vi "extract_offset.vi"(8 "error in (no error)":errorcluster, 10 "xml header string":string, 11 "xpaths":T1) -> (0 "error out":errorcluster, 3 "offset":refnum<class "SpaceVector.lvclass">)   [LabVIEW 2010, in "XImage.xctl"]
uses:
  XImage.xctl
  xpath_cluster.ctl
  classes/SpaceVector/SpaceVector/SpaceVector.lvclass
  classes/XMLElement/XMLElement/XMLElement.lvclass
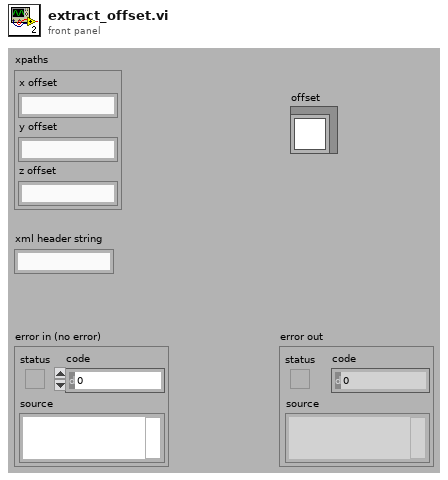
[diagram p1: front panel]
types:
  T1 = typedef "XImage.xctl/xpath_cluster.ctl" = cluster{"x offset":string, "y offset":string, "z offset":string}
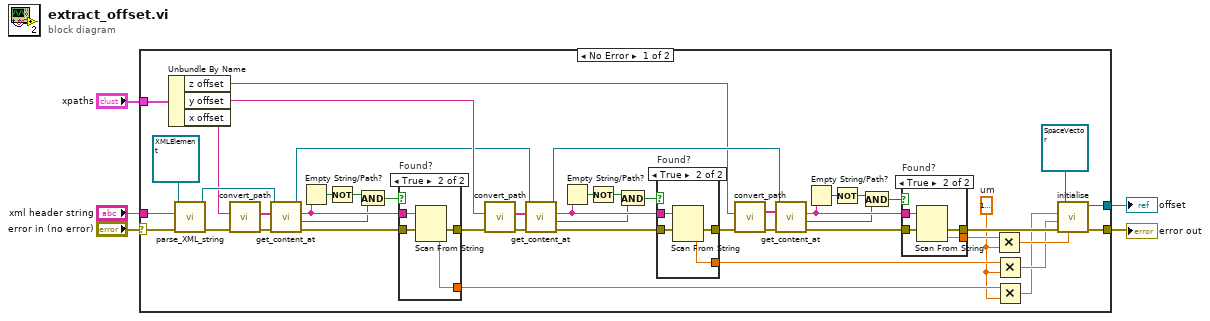
[diagram p0: block diagram]
diagram:
  n1 = case shown="No Error" "error in (no error)" {
    selector: "error in (no error)" -> [w48 w69]
    tunnel: "xml header string" -> [w47 _]
    tunnel: "xpaths" -> [w46 _]
    tunnel: [w32 w69] -> w2
    tunnel: [w30 _] -> w1
    frame No Error {
      w26 = dbl[unit] 1e-06  # um
      n2 = Unbundle By Name(w46) -> ("z offset"=w21:string, "y offset"=w41:string, "x offset"=w22:string)
      n3 = call "parse_XML_string.vi"("error in (no error)"=w48, "XML string"=w47, "Element in"=refnum<class "XMLElement.lvclass"> refnum ("XMLElement.lvclass")) -> ("error out"=w49:errorcluster, "Element out"=w51:refnum<class "XMLElement.lvclass">)  [unwired: 7 in]
      n4 = call "convert_path.vi"("error in (no error)"=w49, "xpath in"=w22) -> ("error out"=w53:errorcluster, "key array out"=w52:string[])  [unwired: 7 in, 1 out]
      n5 = call "get_content_at.vi"("error in (no error)"=w53, "key chain"=w52, "Element in"=w51) -> ("error out"=w38:errorcluster, "found?"=w18:bool, "string"=w20:string, "Element out"=w40:refnum<class "XMLElement.lvclass">)  [unwired: 5 in]
      n6 = Empty String/Path?(string/path=w20) -> (empty?=w19:bool)
      n7 = Not(x=w19) -> (.not. x?=w16:bool)
      n8 = And(x=w16, y=w18) -> (x .and. y?=w17:bool)
      n9 = case "Found?" shown="True" w17 {
        tunnel: w20 -> [_ w68]
        tunnel: w38 -> [w64 w67]
        tunnel: [w64 w66] -> w37
        tunnel: [_ w65] -> w27
        frame False {
        }
        frame True {
          n10 = Scan From String(input string=w68, error in=w67) -> (error out=w66:errorcluster, output 1=w65:dbl)  [unwired: 3 in, 2 out]
        }
      }
      n11 = call "convert_path.vi"("error in (no error)"=w37, "xpath in"=w41) -> ("error out"=w44:errorcluster, "key array out"=w45:string[])  [unwired: 7 in, 1 out]
      n12 = call "get_content_at.vi"("error in (no error)"=w44, "key chain"=w45, "Element in"=w40) -> ("error out"=w36:errorcluster, "found?"=w12:bool, "string"=w13:string, "Element out"=w39:refnum<class "XMLElement.lvclass">)  [unwired: 5 in]
      n13 = Empty String/Path?(string/path=w13) -> (empty?=w14:bool)
      n14 = Not(x=w14) -> (.not. x?=w15:bool)
      n15 = And(x=w15, y=w12) -> (x .and. y?=w11:bool)
      n16 = case "Found?" shown="True" w11 {
        tunnel: w13 -> [_ w63]
        tunnel: w36 -> [w59 w62]
        tunnel: [w59 w61] -> w35
        tunnel: [_ w60] -> w29
        frame False {
        }
        frame True {
          n17 = Scan From String(input string=w63, error in=w62) -> (error out=w61:errorcluster, output 1=w60:dbl)  [unwired: 3 in, 2 out]
        }
      }
      n18 = call "convert_path.vi"("error in (no error)"=w35, "xpath in"=w21) -> ("error out"=w43:errorcluster, "key array out"=w42:string[])  [unwired: 7 in, 1 out]
      n19 = call "get_content_at.vi"("error in (no error)"=w43, "key chain"=w42, "Element in"=w39) -> ("error out"=w34:errorcluster, "found?"=w7:bool, "string"=w8:string)  [unwired: 5 in, 1 out]
      n20 = Empty String/Path?(string/path=w8) -> (empty?=w10:bool)
      n21 = Not(x=w10) -> (.not. x?=w9:bool)
      n22 = And(x=w9, y=w7) -> (x .and. y?=w6:bool)
      n23 = case "Found?" shown="True" w6 {
        tunnel: w8 -> [_ w58]
        tunnel: w34 -> [w54 w57]
        tunnel: [w54 w56] -> w31
        tunnel: [_ w55] -> w28
        frame False {
        }
        frame True {
          n24 = Scan From String(input string=w58, error in=w57) -> (error out=w56:errorcluster, output 1=w55:dbl)  [unwired: 3 in, 2 out]
        }
      }
      n25 = Multiply(x=w28, y=w26) -> (x*y=w25:dbl[unit])
      n26 = Multiply(x=w29, y=w26) -> (x*y=w24:dbl[unit])
      n27 = Multiply(x=w27, y=w26) -> (x*y=w23:dbl[unit])
      n28 = call "initialise.vi"("z"=w25, "error in (no error)"=w31, "y"=w24, "x"=w23, "SpaceVector in"=refnum<class "SpaceVector.lvclass"> refnum ("SpaceVector.lvclass")) -> ("error out"=w32:errorcluster, "SpaceVector out"=w30:refnum<class "SpaceVector.lvclass">)  [unwired: 5 in]
    }
    frame Error {
    }
  }
  "error out" <- w2
  "offset" <- w1
